vi "SV TDMS Write Waveform Unit Info.vi"(0 "tdms file":refnum<k34>, 1 "unit info":T1, 5 "group name":string, 7 "channel name":string, 11 "error in (no error)":errorcluster) -> (4 "tdms file out":refnum<k34>, 6 "group name out":string, 8 "channel name out":string, 15 "error out":errorcluster)   [LabVIEW 2017]
uses:
  <vilib>/addons/_NISVFA/_Shared subVIs/Controls/svc_Unit Info.ctl
  <vilib>/addons/_NISVFA/_Shared subVIs/Controls/NI Channel Properties.ctl
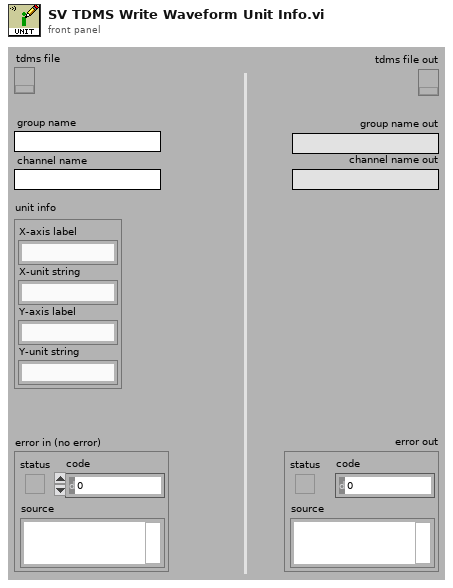
[diagram p1: front panel]
types:
  T1 = typedef "svc_Unit Info.ctl" = cluster{"X-axis label":string, "X-unit string":string, "Y-axis label":string, "Y-unit string":string}
  T2 = typedef "NI Channel Properties.ctl" = u16
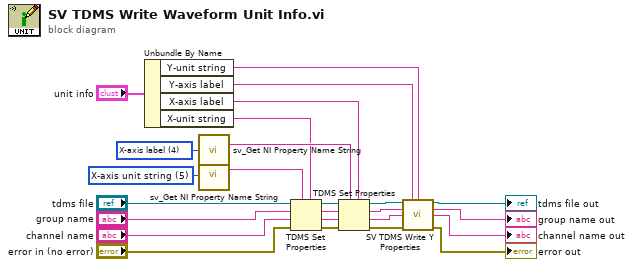
[diagram p0: block diagram]
diagram:
  w20 = T2 5 items=["Channel name", "Channel description", "Y-axis label", "Y-axis unit string", "X-axis label", "X-axis unit string", "x0", "dx", "Number of samples", "X channel", "Filter settled", "dB reference", "Window", "Window parameter", "Window size", "FFT size", "Peak units", "Spectrum type", "Magnitude scale", "Spectral density", "Sensor sensitivity (mV/EU)", "X-axis domain", "LabVIEW datatype"] ("property")
  w21 = T2 4 items=["Channel name", "Channel description", "Y-axis label", "Y-axis unit string", "X-axis label", "X-axis unit string", "x0", "dx", "Number of samples", "X channel", "Filter settled", "dB reference", "Window", "Window parameter", "Window size", "FFT size", "Peak units", "Spectrum type", "Magnitude scale", "Spectral density", "Sensor sensitivity (mV/EU)", "X-axis domain", "LabVIEW datatype"] ("property")
  n1 = Unbundle By Name("unit info") -> ("Y-unit string"=w1:string, "Y-axis label"=w7:string, "X-axis label"=w15:string, "X-unit string"=w16:string)
  n2 = call <vilib>:"sv_Get NI Property Name String.vi"("property"=w21) -> ("TDMS property name"=w18:string)  [unwired: 13 in, 1 out]
  n3 = call <vilib>:"sv_Get NI Property Name String.vi"("property"=w20) -> ("TDMS property name"=w19:string)  [unwired: 13 in, 1 out]
  n4 = TDMS Set Properties(5:w16, 7:w19, 8:"error in (no error)", 9:"channel name", 10:"group name", 11:"tdms file") -> (0:w25:errorcluster, 1:w24:string, 2:w23:string, 3:w22:refnum<k34>)
  n5 = TDMS Set Properties(5:w15, 7:w18, 8:w25, 9:w24, 10:w23, 11:w22) -> (0:w3:errorcluster, 1:w8:string, 2:w2:string, 3:w10:refnum<k34>)
  n6 = call <vilib>:"SV TDMS Write Y Properties.vi"("tdms file"=w10, "y-axis label"=w7, "y-unit string"=w1, "group name"=w2, "channel name"=w8, "error in (no error)"=w3) -> ("tdms file out"=→"tdms file out":refnum<k34>, "group name"=→"group name out":string, "channel name"=→"channel name out":string, "error out"=→"error out":errorcluster)  [unwired: 6 in]
